vi "svx_Extract Segment (Rev).vi"(6 "indice":cluster{"start":i32, "length":i32}, 7 "reset?":bool, 8 "old end reached":bool, 9 "end reached":bool, 10 "data in":dbl[](array[numeric]), 11 "old order data":dbl[](array[numeric])) -> (0 "end reached out":bool, 2 "data out":dbl[](array[numeric]), 3 "remaining data":dbl[](array[numeric]))   [LabVIEW 2017]
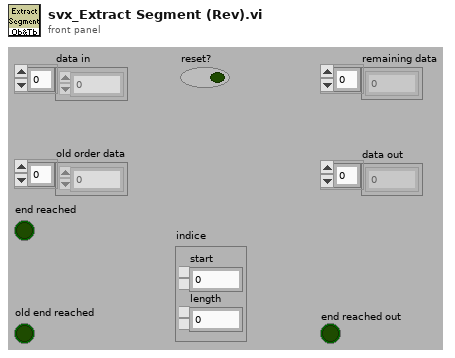
[diagram p1: front panel]
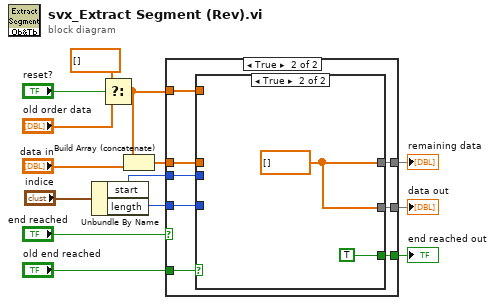
[diagram p0: block diagram]
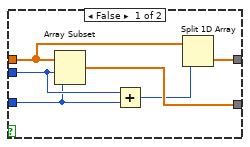
[diagram p2: hidden frame]
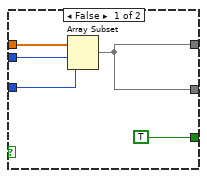
[diagram p3: hidden frame]
diagram:
  n1 = Unbundle By Name("indice") -> ("start"=w2:i32, "length"=w1:i32)
  n2 = Select(t=dbl[] [], s="reset?", f="old order data") -> (s? t:f=w12:dbl[])
  n3 = Build Array (concatenate)(w12, "data in") -> (w13:dbl[])
  n4 = case shown="True" "end reached" {
    tunnel: w13 -> [w18 w23]
    tunnel: w12 -> [_ w24]
    tunnel: [w20 w26] -> w6
    tunnel: [_ w28] -> w4
    tunnel: "old end reached" -> [_ w27]
    tunnel: [w19 w25] -> w5
    tunnel: w2 -> [w17 w22]
    tunnel: w1 -> [w16 w21]
    frame False {
      n5 = Array Subset(array=w18, index=w17, length=w16) -> (w19:dbl[])
      n6 = Add(x=w17, y=w16) -> (x+y=w15:i32)
      n7 = Split 1D Array(array=w18, index=w15) -> (second subarray=w20:dbl[])  [unwired: 1 out]
    }
    frame True {
      n8 = case shown="True" w27 {
        tunnel: [TRUE ("end reach?") TRUE ("end reach?")] -> w28
        tunnel: w21 -> [w30 _]
        tunnel: [w29 w34] -> w26
        tunnel: [w29 w34] -> w25
        tunnel: w24 -> [_ _]
        tunnel: w23 -> [w32 _]
        tunnel: w22 -> [w31 _]
        frame False {
          n9 = Array Subset(array=w32, index=w31, length=w30) -> (w29:dbl[])
        }
        frame True {
          w34 = dbl[] [] ("old order data")
        }
      }
    }
  }
  "remaining data" <- w6
  "data out" <- w5
  "end reached out" <- w4
